vi "Configure Comparator.vi"(0 "VISA resource name":refnum<visa-resource-name>, 1 "Upper Limit (0.0)":dbl min=-1e+27 max=9.99999e+26 step=1e-15 format="%_6g", 5 "Enable Calculate Comparator  (F: Disable)":bool, 9 "Comparator Beeper  (0: Off)":u16(ring) format="%_1g" items=["Off", "High", "Go", "Low", "High or Low"], 11 "error in (no error)":errorcluster, 12 "Lower Limit (0.0)":dbl min=-9.99999e+26 max=9.99999e+26 step=1e-15 format="%_6g") -> (4 "VISA resource name out":refnum<visa-resource-name>, 15 "error out":errorcluster)   [LabVIEW 2017, in "ADCMT 6240.lvlib"]
doc: "This VI configures the comparator calculation.\n\n<B>Note:</B> Operation is not performed in a burst mode."
uses:
  ADCMT 6240.lvlib
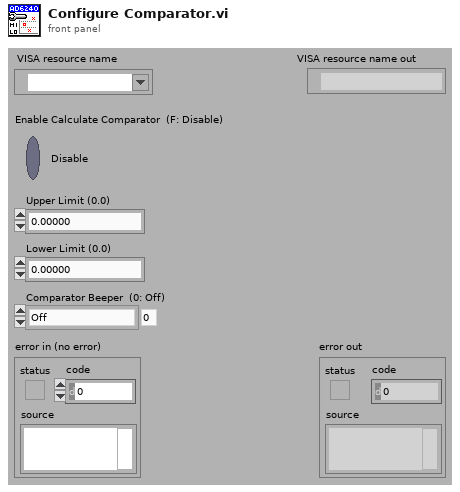
[diagram p1: front panel]
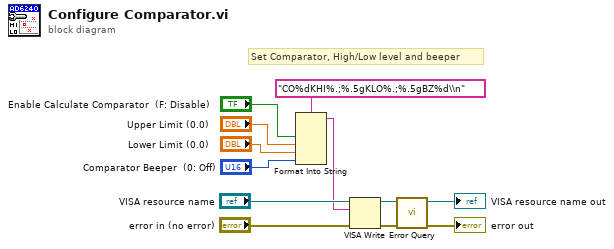
[diagram p0: block diagram]
diagram:
  # "Set Comparator, High/Low level and beeper"
  n1 = Format Into String(format string="CO%dKHI%.;%.5gKLO%.;%.5gBZ%d\\n" ("Limit Lower"), "Enable Calculate Comparator  (F: Disable)", "Upper Limit (0.0)", "Lower Limit (0.0)", "Comparator Beeper  (0: Off)") -> (resulting string=w4:string)  [unwired: 2 in, 1 out]
  n2 = VISA Write(VISA resource name="VISA resource name", write buffer=w4, error in (no error)="error in (no error)") -> (VISA resource name out=w8:refnum<visa-resource-name>, error out=w7:errorcluster)  [unwired: 1 out]
  n3 = call "Error Query.vi"("error in (no error)"=w7, "VISA resource name"=w8) -> ("error out"=→"error out":errorcluster, "VISA resource name out"=→"VISA resource name out":refnum<visa-resource-name>)  [unwired: 6 in, 2 out]
